vi "logo Address.vi"(9 "path":path) -> (1 "字符串":string)   [LabVIEW 2014]
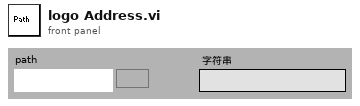
[diagram p1: front panel]
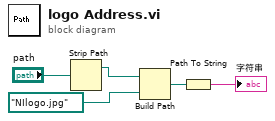
[diagram p0: block diagram]
diagram:
  n1 = Strip Path(path="path") -> (stripped path=w2:path)  [unwired: 1 out]
  n2 = Build Path(base path=w2, name or relative path=path "NIlogo.jpg") -> (appended path=w4:path)
  n3 = Path To String(path=w4) -> (string=→"字符串":string)
